vi "GV FIFOin finished.vi"() -> ()   [LabVIEW 2017]
panel:
  in  "FIFOin finished":bool
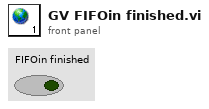
[diagram p1: front panel]
diagram:
